vi "create swap encoder command.vi"(10 "swap encoders":bool=TRUE) -> (3 "command message":variant)   [LabVIEW 2018, in "RT - FPGA commands.lvlib"]
uses:
  RT - FPGA commands.lvlib
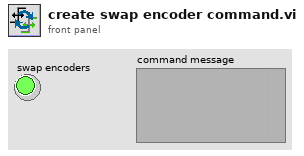
[diagram p1: front panel]
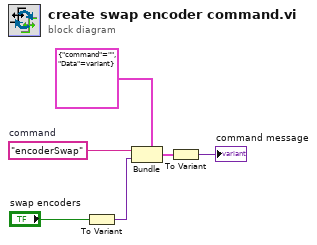
[diagram p0: block diagram]
diagram:
  w5 = "encoderSwap"  # command
  n1 = To Variant(anything="swap encoders") -> (Variant=w4:variant)
  n2 = Bundle(cluster=cluster{"command":string, "Data":variant} {"command"="", "Data"=variant}, "command"=w5, "Data"=w4) -> (w3:cluster{"command":string, "Data":variant})
  n3 = To Variant(anything=w3) -> (Variant=→"command message":variant)
